vi "HandleServo.vi"(11 "DPadValue":dbl) -> (3 "Action":T1)   [LabVIEW 2015]
doc: "Determines what action the servo should take based on the Dpad input. Dpad is rounded to the nearest integer, and the integers correspond to these states:\n0: Disable\n1: Raise\n-1: Lower"
uses:
  ServoAction.ctl
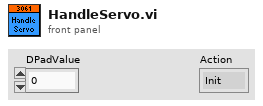
[diagram p1: front panel]
types:
  T1 = typedef "ServoAction.ctl" = enum16{"Init", "SetAngle", "GetAngle", "Lower", "Raise", "Disable"}
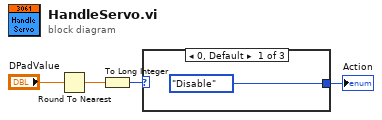
[diagram p0: block diagram]
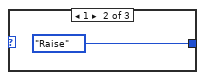
[diagram p2: hidden frame]
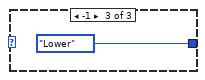
[diagram p3: hidden frame]
diagram:
  n1 = Round To Nearest(number="DPadValue") -> (nearest integer value=w1:dbl)
  n2 = To Long Integer(number=w1) -> (32bit integer=w3:i32)
  n3 = case shown="0, Default" w3 {
    tunnel: [ServoAction."Disable" ("Action") ServoAction."Raise" ("Action") ServoAction."Lower" ("Action")] -> w2
    frame 0, Default {
    }
    frame 1 {
    }
    frame -1 {
    }
  }
  "Action" <- w2
